vi "JsonToParameterClass.vi"(8 "error in (no error)":errorcluster, 11 "JSON String":string) -> (0 "error out":errorcluster, 3 "Parameter Out":refnum<class "Parameter.lvclass">)   [LabVIEW 2023, in "Easy.SequenceManagerLabVIEW.lvlib" / "Parameter.lvclass"]
uses:
  Parameter.lvclass
  <vilib>/G Craftsman/JSON Object Serialization/JSON Object Serialization/GCraftsman JSON Serialization/GCraftsman JSON Serialization.lvlib
panel:
  # "Connector Pane"
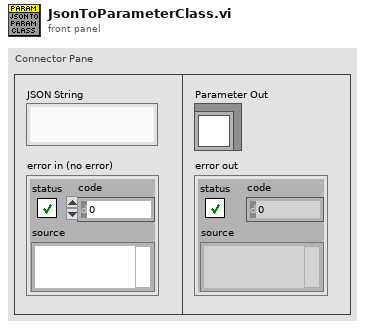
[diagram p1: front panel]
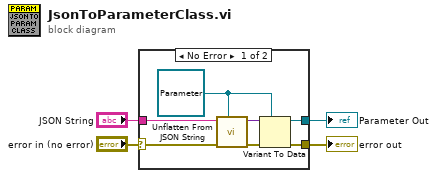
[diagram p0: block diagram]
diagram:
  n1 = case shown="No Error" "error in (no error)" {
    selector: "error in (no error)" -> [w7 w12]
    tunnel: [w9 w12] -> w3
    tunnel: "JSON String" -> [w6 _]
    tunnel: [w5 _] -> w1
    frame No Error {
      w10 = refnum<class "Parameter.lvclass"> refnum ("Easy.SequenceManagerLabVIEW.lvlib:Parameter.lvclass")
      n2 = call <vilib>:"Unflatten From JSON String.vi"("Type and Defaults"=w10, "error in (no error)"=w7, "JSON String"=w6) -> ("error out"=w8:errorcluster, "Variant"=w11:variant)  [unwired: 7 in]
      n3 = Variant To Data(error in=w8, type=w10, Variant=w11) -> (data=w5:refnum<class "Parameter.lvclass">, error out=w9:errorcluster)
    }
    frame Error {
    }
  }
  "error out" <- w3
  "Parameter Out" <- w1
